vi "Configure the Function on 2nd Display.vi"(5 "Manual Range":dbl format="%#.9e", 7 "Enable Auto Range":bool=TRUE, 8 "error in":errorcluster, 10 "Function":u8(ring)=7 items=["DC Voltage", "AC Voltage", "DC Current", "AC Current", "2-Wire Resistance", "Frequency", "Period", "None"], 11 "VISA resource name":refnum<visa-resource-name>) -> (0 "error out":errorcluster, 3 "VISA resource name out":refnum<visa-resource-name>)   [LabVIEW 2011, in "DMM4.lvlib"]
uses:
  <instrlib>/DMM4/DMM4.lvlib
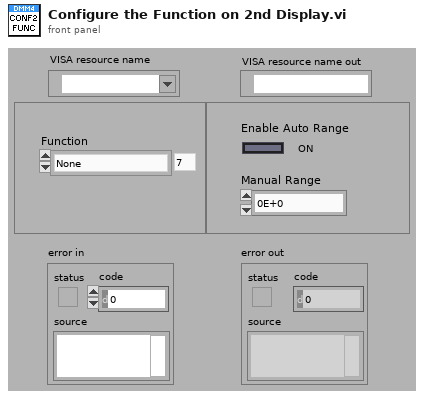
[diagram p1: front panel]
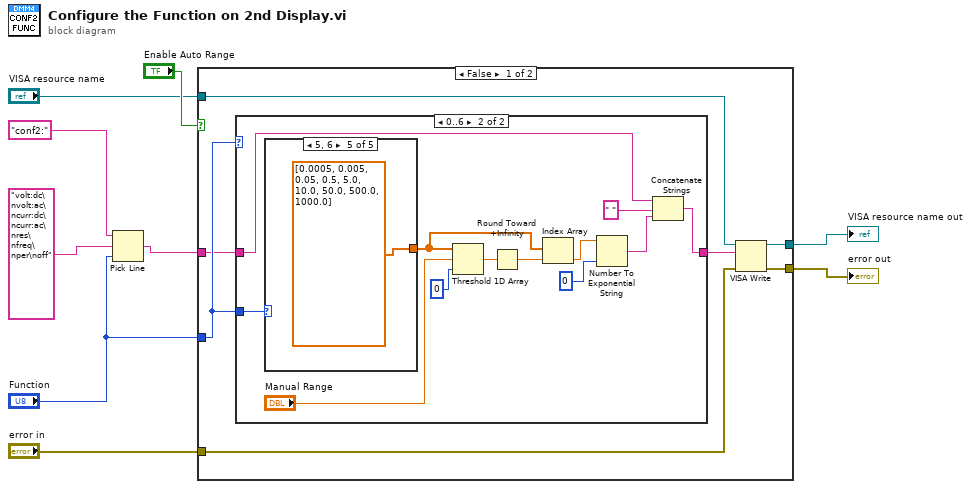
[diagram p0: block diagram]
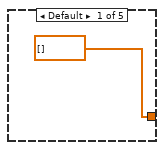
[diagram p3: hidden frame]
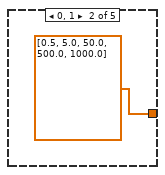
[diagram p4: hidden frame]
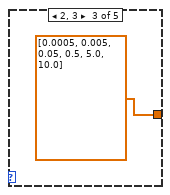
[diagram p5: hidden frame]
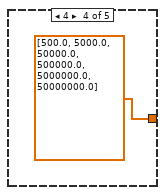
[diagram p6: hidden frame]
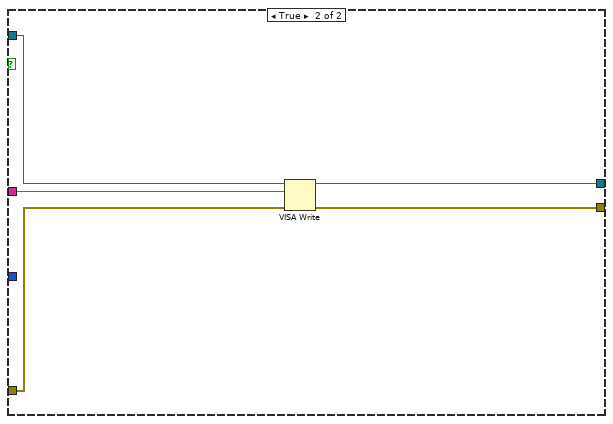
[diagram p7: hidden frame]
diagram:
  n1 = Pick Line(string ("")="conf2:", multi-line string="volt:dc\nvolt:ac\ncurr:dc\ncurr:ac\nres\nfreq\nper\noff", line index="Function") -> (output string=w5:string)
  n2 = case shown="False" "Enable Auto Range" {
    tunnel: "Function" -> [w16 _]
    tunnel: w5 -> [w15 w39]
    tunnel: "VISA resource name" -> [w13 w38]
    tunnel: "error in" -> [w12 w37]
    tunnel: [w11 w36] -> w2
    tunnel: [w10 w35] -> w1
    frame False {
      n3 = case shown="0..6" w16 {
        tunnel: w16 -> [_ w18]
        tunnel: w15 -> [w17 w20]
        tunnel: [w17 w19] -> w14
        frame Default {
        }
        frame 0..6 {
          n4 = case shown="5, 6" w18 {
            tunnel: [dbl[] [] dbl[] [0.5, 5.0, 50.0, 500.0, 1000.0] dbl[] [0.0005, 0.005, 0.05, 0.5, 5.0, 10.0] dbl[] [500.0, 5000.0, 50000.0, 500000.0, 5000000.0, 50000000.0] dbl[] [0.0005, 0.005, 0.05, 0.5, 5.0, 10.0, 50.0, 500.0, 1000.0]] -> w25
            frame Default {
            }
            frame 0, 1 {
            }
            frame 2, 3 {
            }
            frame 4 {
            }
            frame 5, 6 {
            }
          }
          n5 = Threshold 1D Array(1:0 ("start index (0)"), 2:"Manual Range", 3:w25) -> (0:w27:dbl)
          n6 = Round Toward +Infinity(x=w27) -> (ceil(x): smallest int >= x=w26:dbl)
          n7 = Index Array(array=w25, index=w26) -> (element=w24:dbl)
          n8 = Number To Exponential String(number=w24, precision (6)=i16 0) -> (E-format string=w21:string)  [unwired: 2 in]
          n9 = Concatenate Strings(w20, " " ("string"), w21) -> (w19:string)
        }
      }
      n10 = VISA Write(VISA resource name=w13, write buffer=w14, error in (no error)=w12) -> (VISA resource name out=w11:refnum<visa-resource-name>, error out=w10:errorcluster)  [unwired: 1 out]
    }
    frame True {
      n11 = VISA Write(VISA resource name=w38, write buffer=w39, error in (no error)=w37) -> (VISA resource name out=w36:refnum<visa-resource-name>, error out=w35:errorcluster)  [unwired: 1 out]
    }
  }
  "VISA resource name out" <- w2
  "error out" <- w1
